vi "Disconnect from Server.vi"(8 "error in (no error)":errorcluster, 11 "Client in":refnum<class "Client.lvclass">) -> (0 "error out":errorcluster, 1 "timed out":bool, 3 "Client out":refnum<class "Client.lvclass">)   [LabVIEW 2013, in "MQTT Server.lvlib" / "Client.lvclass"]
uses:
  Client.lvclass
  Client.lvclass/Client.ctl
  Control Packets/DISCONNECT/DISCONNECT.lvclass
  Server/Session/Session.lvclass
  Server/Connection/TCPConnection.lvclass
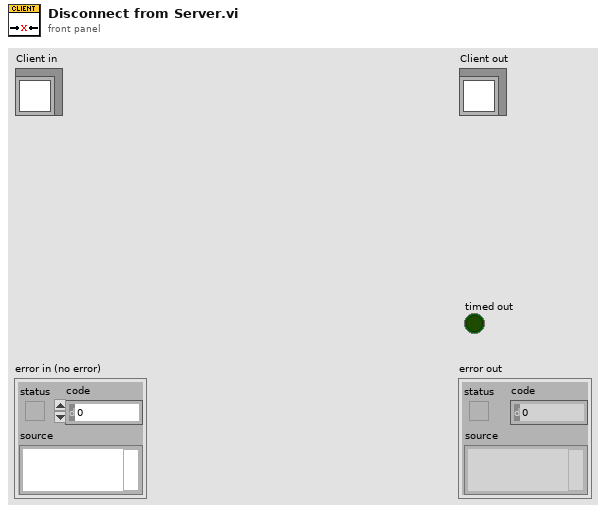
[diagram p1: front panel]
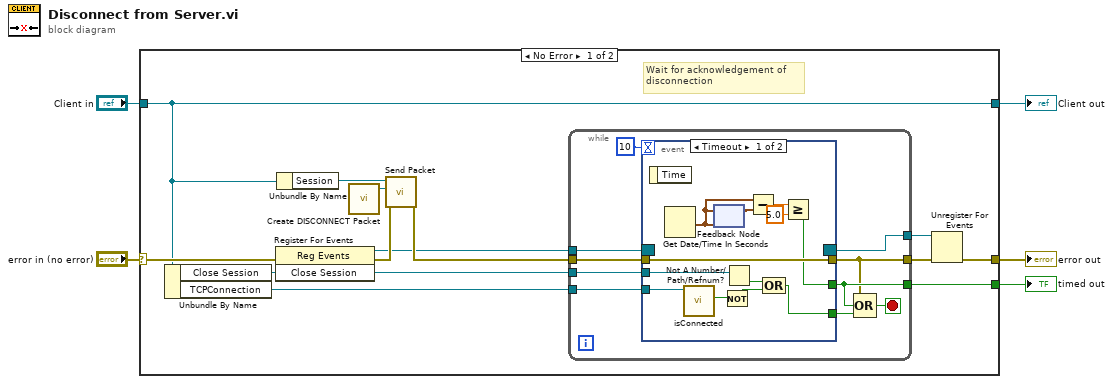
[diagram p0: block diagram]
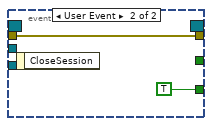
[diagram p2: hidden frame]
diagram:
  n1 = case shown="No Error" "error in (no error)" {
    selector: "error in (no error)" -> [w18 w44]
    tunnel: [w17 w44] -> w4
    tunnel: [w7 w43] -> w2
    tunnel: "Client in" -> [w7 w43]
    tunnel: [w16 _] -> w1
    frame No Error {
      # "Wait for acknowledgement of\ndisconnection"
      n2 = Unbundle By Name(w7) -> ("Close Session"=w6:refnum<user-event>, "TCPConnection"=w8:refnum<class "TCPConnection.lvclass">)
      n3 = register-events(error in=w18, w6) -> (reference out=w9:refnum<event-registration>, error out=w13:errorcluster)  [unwired: 1 in]
      n4 = Unbundle By Name(w7) -> ("Session"=w15:refnum<class "Session.lvclass">)
      n5 = call "Create DISCONNECT Packet.vi"() -> ("DISCONNECT"=w14:refnum<class "DISCONNECT.lvclass">)  [unwired: 10 in, 1 out]
      n6 = call "Send Packet.vi"("error in (no error)"=w13, "Packet"=w14, "Session in"=w15) -> ("error out"=w10:errorcluster)  [unwired: 5 in, 3 out]
      n7 = while {
        tunnel: [w22] -> w16
        tunnel: [w28] -> w12
        tunnel: [w21] -> w11
        tunnel: w10 -> [w27]
        tunnel: w9 -> [w26]
        tunnel: w8 -> [w20]
        tunnel: w6 -> [w19]
        stop <- w23 stop-if-true
        n8 = event shown="[0] Timeout" {
          selector: w26 -> [_ _]
          dyn-events: [_ _] -> w28
          timeout: 10 -> [_ _]
          tunnel: [w40 w42] -> w21
          tunnel: w27 -> [w40 w42]
          tunnel: [w34 _] -> w22
          tunnel: [w29 TRUE] -> w24
          tunnel: w20 -> [w39 _]
          tunnel: w19 -> [w32 _]
          event Timeout {
            n9 = event-data() -> ()  [unwired: 1 in, 1 out]
            n10 = Get Date/Time In Seconds() -> (seconds since 1Jan1904=w37:timestamp)
            n11 = call "isConnected.vi"("TCPConnection in"=w39) -> ("connected"=w33:bool)  [unwired: 8 in, 2 out]
            n12 = feedback #1(w37) -> (w38:timestamp)
            n13 = feedback-in #1(w37) -> ()
            n14 = Not(x=w33) -> (.not. x?=w30:bool)
            n15 = Not A Number/Path/Refnum?(number/path/refnum=w32) -> (NaN/Path/Refnum?=w31:bool)
            n16 = Subtract(x=w37, y=w38) -> (x-y=w36:dbl)
            n17 = Compound Arithmetic op=OR(w31, w30) -> (w29:bool)
            n18 = Greater Or Equal?(x=w36, y=5.0) -> (x >= y?=w34:bool)
          }
          event User Event {
            n19 = event-data() -> ()  [unwired: 1 in, 1 out]
          }
        }
        n20 = Compound Arithmetic op=OR(w21, w22, w24) -> (w23:bool)
      }
      n21 = Unregister For Events(event registration refnum=w12, error in=w11) -> (error out=w17:errorcluster)
    }
    frame Error {
    }
  }
  "error out" <- w4
  "Client out" <- w2
  "timed out" <- w1
